vi "Check_running.vi"(8 "error in (no error)":errorcluster, 11 "Lifter_motor in":refnum<class "Lifter_motor.lvclass">) -> (0 "error out":errorcluster, 1 "Motor Status":string, 2 "Status":bool, 3 "Lifter_motor out":refnum<class "Lifter_motor.lvclass">)   [LabVIEW 2019, in "Lifter_motor.lvclass"]
uses:
  Lifter_motor.lvclass
  Lifter_motor.lvclass/Lifter_motor.ctl
  TCP Class/LifterTCP.lvclass
panel:
  out "Velocity":dbl
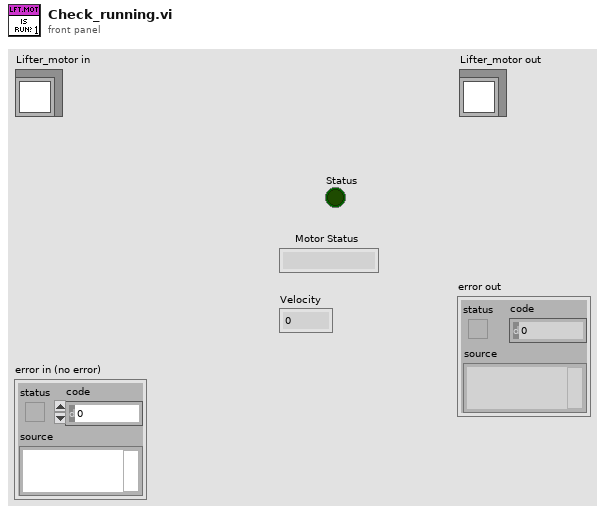
[diagram p1: front panel]
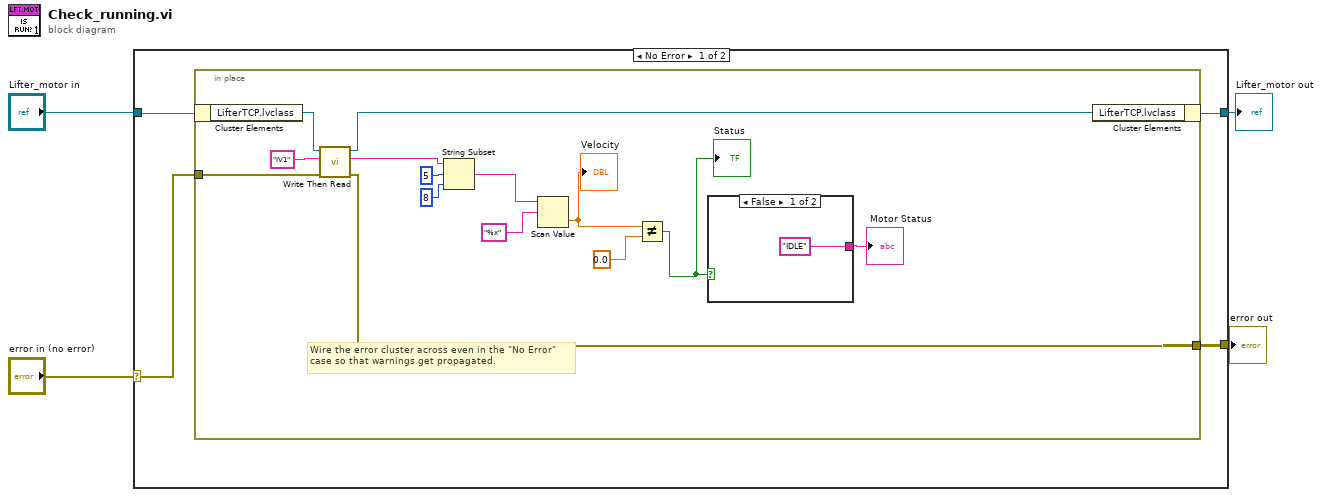
[diagram p0: block diagram]
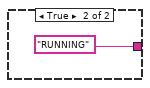
[diagram p2: hidden frame]
diagram:
  n1 = case shown="No Error" "error in (no error)" {
    selector: "error in (no error)" -> [w7 w26]
    tunnel: [w6 w26] -> w3
    tunnel: [w5 w25] -> w1
    tunnel: "Lifter_motor in" -> [w8 w25]
    frame No Error {
      # "Wire the error cluster across even in the \"No Error\"\ncase so that warnings get propagated."
      n2 = in-place {
        in-place-border: w7 -> [w21]
        in-place-border: [w9] -> w6
        n3 = in-place-cluster #1(w8) -> ("LifterTCP.lvclass"=w22:refnum<class "LifterTCP.lvclass">)
        n4 = call "Write Then Read.vi"("error in (no error)"=w21, "Parameter 1"="IV1", "LifterTCP in"=w22) -> ("error out"=w9:errorcluster, "Read Data"=w17:string, "LifterTCP out"=w20:refnum<class "LifterTCP.lvclass">)  [unwired: 6 in]
        n5 = String Subset(string=w17, offset (0)=5, length (rest)=8 ("length (rest)")) -> (substring=w10:string)
        n6 = Scan Value(string=w10, format string="%x") -> (value=w14:dbl)  [unwired: 1 in, 1 out]
        "Velocity" <- w14
        n7 = Not Equal?(x=w14, y=0.0) -> (x != y?=w12:bool)
        "Status" <- w12
        n8 = case shown="False" w12 {
          tunnel: ["IDLE" ("Motor") "RUNNING" ("Motor")] -> w11
          frame False {
          }
          frame True {
          }
        }
        "Motor Status" <- w11
        n9 = in-place-cluster #1("LifterTCP.lvclass"=w20) -> (w5:refnum<class "Lifter_motor.lvclass">)
      }
    }
    frame Error {
    }
  }
  "error out" <- w3
  "Lifter_motor out" <- w1
